vi "RefMem PtByPt RT Driver VI (Async).vi"(6 "Device Clock":string, 9 "Device Inputs FIFO":refnum<k33>, 10 "Device Outputs FIFO":refnum<k33>, 11 "Device Reference":T1 format="%.0x") -> ()   [LabVIEW 2010, in "RefMem PtByPt Custom Device.lvlib"]
uses:
  RefMem PtByPt Custom Device.lvlib
  <vilib>/NI Veristand/Custom Device API/Custom Device Item Ref.ctl
  <vilib>/NI Veristand/Custom Device API/Custom Device Channel Type.ctl
  Controls/Data Channel Type.ctl
  <vilib>/Platform/TimedLoop/XDataNode/XDataNode.xnode
  <vilib>/Platform/TimedLoop/XDataNode/timing_clust.ctl
  <vilib>/Platform/TimedLoop/XDataNode/nitl_modes.ctl
  <vilib>/Platform/TimedLoop/XDataNode/wakeup.ctl
  Controls/Global.vi
  <vilib>/NI Veristand/Custom Device API/Get Item Property (I32).vi
  <vilib>/NI Veristand/Custom Device API/Get Item Property (String).vi
  <vilib>/NI Veristand/Custom Device Tools/Custom Device Utility Library/NI VeriStand - Search for All Items by Property.vi
  <vilib>/NI Veristand/Custom Device API/Get Item Property (U32).vi
  <vilib>/NI Veristand/Custom Device Tools/Custom Device Utility Library/NI VeriStand - Search for Item by Name.vi
  <vilib>/Platform/TimedLoop/XDataNode/XDNodeRunTimeDep.lvlib
  <vilib>/NI Veristand/Custom Device API/Custom Device API.lvlib
  <vilib>/NI Veristand/Custom Device Tools/Custom Device Utility Library/Custom Device Utility Library.lvlib
panel:
  in  "Status Notifier":refnum<notifier>
  # "Custom Device Template\nv1.0"
  # "Use this template as a starting point for creating a custom device code module. The input controls shown here are specially named controls that the system will use to provide the device loop with data. The controls are not required for the device loop to run. For instance, if the device doesn't produce any output data, then you don't need the Device Outputs FIFO control. If you do use these controls, however, they need to have these exact names to be functional."
  # "The optional status notifier element is used to notify the RT engine of the last state of the custom device, and to indicate the device has completed execution. If this control is not used, a default No Error value is returned to the system when the device finishes execution.\n\nNote: This error state is not checked until the system shuts down. Use an output status channel to send more immediate status values to the system."
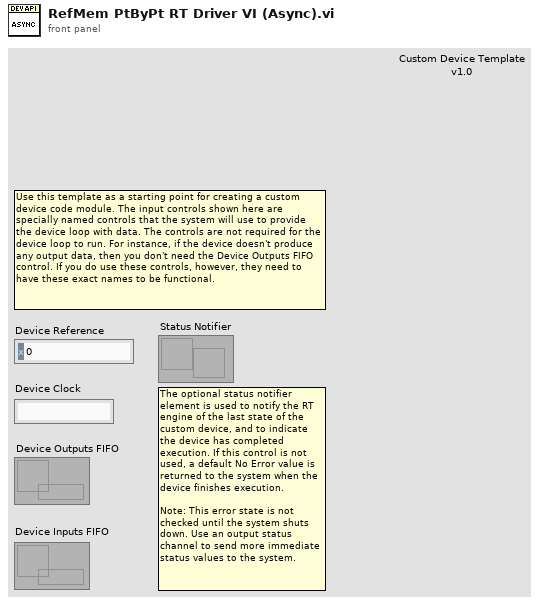
[diagram p1: front panel]
types:
  T1 = typedef "Custom Device API.lvlib/Custom Device Item Ref.ctl" = u64
  T2 = typedef "RefMem PtByPt Custom Device.lvlib/Data Channel Type.ctl" = enum16{"Read", "Write"}
  T3 = typedef "Custom Device API.lvlib/Custom Device Channel Type.ctl" = enum16{"Input", "Output"}
  T4 = typedef "Custom Device API.lvlib/Custom Device Timed Loop Priority.ctl" = enum32{"Low", "Medium", "High"}
  T5 = typedef "XDNodeRunTimeDep.lvlib/timing_clust.ctl" = cluster{"Expected End [f-1]":u64, "Actual End [f-1]":u64, "Finished Late? [f-1]":bool, "Expected End [i-1]":u64, "Actual End [i-1]":u64, "Finished Late? [i-1]":bool, "Expected Start [i]":u64, "Actual Start [i]":u64, "Expected Start [f]":u64, "Actual Start [f]":u64, "Source Name":string, "Structure Name":string, "Period":i64, "Deadline":i64, "Offset":i64, "Start":i64, "Priority":i32, "Timeout":i32, "Mode":T6, "Wakeup Reason":T7, "Error":errorcluster, "Source Type":string, "Secondary Source Type":string, "Global End Time":u64, "Global Start Time":u64, "Frame Duration":u64, "Iteration Duration":u64, "Assigned CPU":i32, "I/O Scan Engine Mode":u32}
  T6 = typedef "XDNodeRunTimeDep.lvlib/nitl_modes.ctl" = enum32{"No Change", "Process missed periods, maintain original phase", "Discard missed periods, maintain original phase", "Process missed periods, ignore original phase", "Discard missed periods, ignore original phase"}
  T7 = typedef "XDNodeRunTimeDep.lvlib/wakeup.ctl" = enum32{"Normal", "Aborted", "Asynchronous wakeup", "Timing source error", "Timed loop error", "Timeout"}
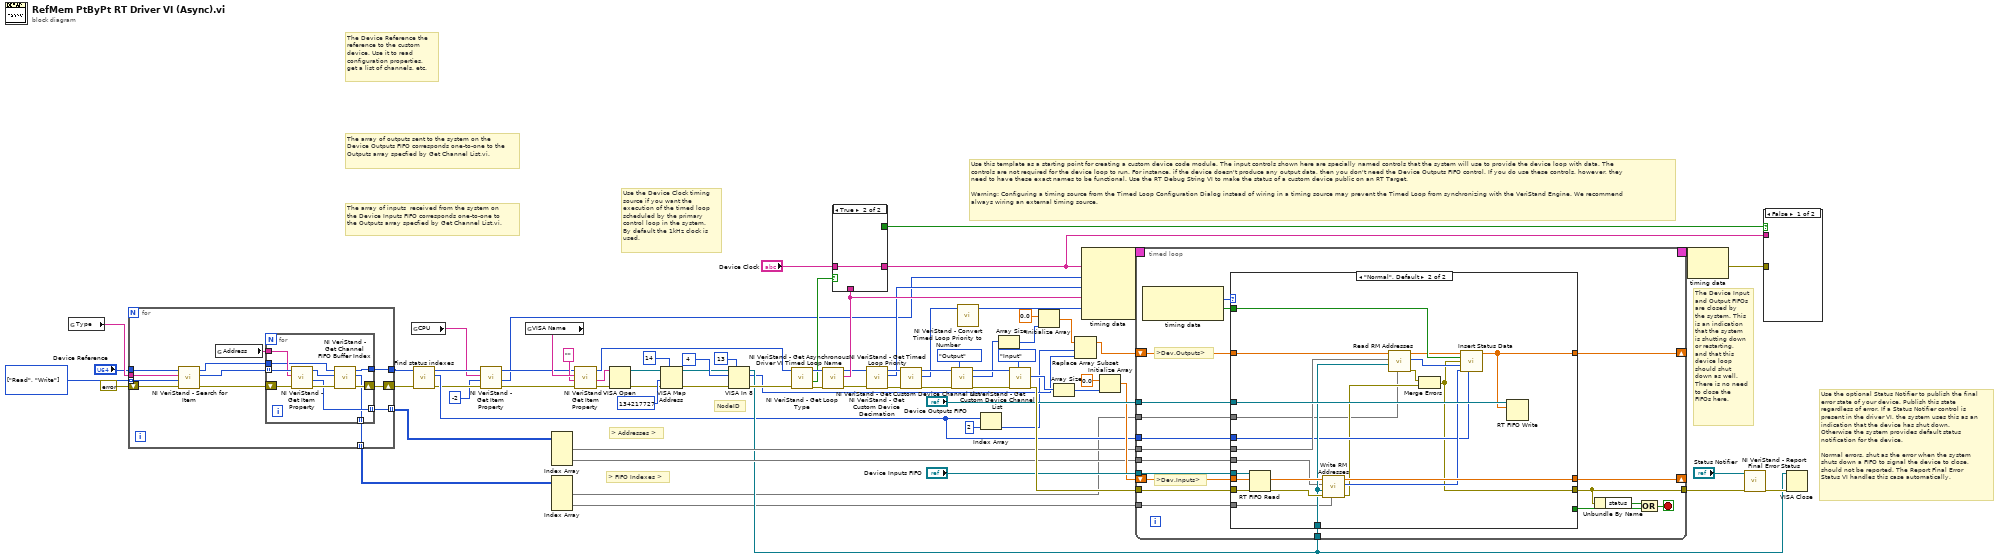
[diagram p0: block diagram]
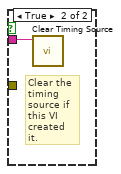
[diagram p2: hidden frame]
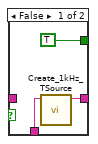
[diagram p3: hidden frame]
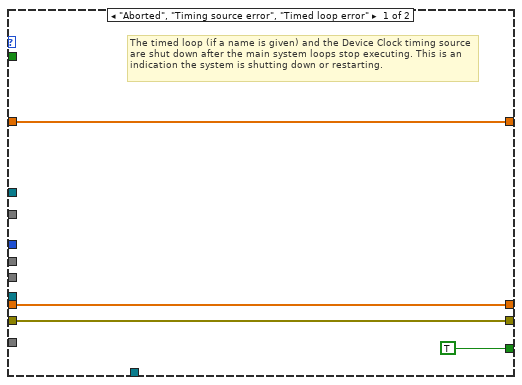
[diagram p4: hidden frame]
diagram:
  w31 = T2[] [enum."Read", enum."Write"] items=["Read", "Write"]
  # "> FIFO Indexes >"
  # "> Addresses >"
  # "NodeID"
  # "The array of inputs  received from the system on the Device Inputs FIFO corresponds one-to-one to the Outputs array specfied by Get Channel List.vi."
  # "Use the optional Status Notifier to publish the final error state of your device. Publish this state regardless of error. If a Status Notifier control is present in the driver VI, the system uses this as an indication that the device has shut down. Otherwise the system provides default status notification for the device.\n\nNormal errors, shut as the error when the system shuts down a FIFO to signal the device to close, should not be reported. The Report Final Error Status VI handles this case automatically."
  # "The Device Input and Output FIFOs are closed by the system. This is an indication that the system is shutting down or restarting, and that this device loop should shut down as well. There is no need to close the FIFOs here."
  # "The array of outputs sent to the system on the Device Outputs FIFO corresponds one-to-one to the Outputs array specfied by Get Channel List.vi."
  # "The Device Reference the reference to the custom device. Use it to read configuration properties, get a list of channels, etc."
  # "Use the Device Clock timing source if you want the execution of the timed loop scheduled by the primary control loop in the system. \nBy default the 1kHz clock is used."
  # "Use this template as a starting point for creating a custom device code module. The input controls shown here are specially named controls that the system will use to provide the device loop with data. The controls are not required for the device loop to run. For instance, if the device doesn't produce any output data, then you don't need the Device Outputs FIFO control. If you do use these controls, however, they need to have these exact names to be functional. Use the RT Debug String VI to make the status of a custom device public on an RT Target.\n\nWarning: Configuring a timing source from the Timed Loop Configuration Dialog instead of wiring in a timing source may prevent the Timed Loop from synchronizing with the VeriStand Engine. We recommend always wiring an external timing source."
  n1 = global read "Global.vi" "Type"() -> (w33:string)
  n2 = for {
    tunnel: w33 -> [w88]
    tunnel: "Device Reference" -> [w87]
    tunnel: w31 -> [w86] mode=indexing
    shift-right: [w81] -> w15
    shift-left: errorcluster {"status"=FALSE, "code"=0, "source"=""} ("error in (no error)") -> [w85]
    tunnel: [w80] -> w29 mode=indexing
    tunnel: [w78] -> w16
    tunnel: [w77] -> w10 mode=indexing
    n3 = call-poly <vilib>:"NI VeriStand - Search for Item.vi"("error in"=w85, "Property Value"=w86, "Property Name"=w88, "Section Ref in"=w87) -> ("error out"=w84:errorcluster, "Item Refs"=w83:T1[], "Section Ref out"=w79:T1)  [unwired: 4 in, 1 out]
    n4 = global read "Global.vi" "Address"() -> (w82:string)
    n5 = for {
      tunnel: w83 -> [w97] mode=indexing
      tunnel: w82 -> [w96]
      shift-right: [w91] -> w81
      shift-left: w84 -> [w98]
      tunnel: [w90] -> w80 mode=indexing
      tunnel: w79 -> [w93]
      tunnel: [w92] -> w78
      tunnel: [w89] -> w77 mode=indexing
      n6 = call-poly <vilib>:"NI VeriStand - Get Item Property.vi"("error in (no error)"=w98, "Property Name"=w96, "Item Ref in"=w97) -> ("error out"=w95:errorcluster, "Value"=w90:u32, "Item Ref out"=w94:T1)  [unwired: 5 in, 1 out]
      n7 = call <vilib>:"NI VeriStand - Get Channel FIFO Buffer Index.vi"("error in"=w95, "Channel Ref"=w94, "Device Ref in"=w93) -> ("error out"=w91:errorcluster, "Channel FIFO Buffer Index"=w89:i32, "Device Ref out"=w92:T1)  [unwired: 4 in, 2 out]
    }
  }
  n8 = global read "Global.vi" "CPU"() -> (w5:string)
  n9 = call "Find status indexes.vi"("error in (no error)"=w15, "Custom Device ref"=w16) -> ("error out"=w6:errorcluster, "Indexes"=w11:i32[], "Custom Device ref"=w7:T1)  [unwired: 7 in]
  n10 = call-poly <vilib>:"NI VeriStand - Get Item Property.vi"("error in (no error)"=w6, "Default Value"=-2 ("Automatic Processor"), "Property Name"=w5, "Item Ref in"=w7) -> ("error out"=w3:errorcluster, "Value"=w1:i32, "Item Ref out"=w2:T1)  [unwired: 4 in, 1 out]
  n11 = global read "Global.vi" "VISA Name"() -> (w43:string)
  n12 = Index Array(array=w29) -> (element #1=w28:u32[], element #2=w27:u32[])  [unwired: 4 in]
  n13 = Index Array(array=w10) -> (element #1=w8:i32[], element #2=w9:i32[])  [unwired: 4 in]
  n14 = call-poly <vilib>:"NI VeriStand - Get Item Property.vi"("error in (no error)"=w3, "Default Value"="", "Property Name"=w43, "Item Ref in"=w2) -> ("error out"=w38:errorcluster, "Value"=w37:string, "Item Ref out"=w35:T1)  [unwired: 4 in, 1 out]
  n15 = VISA Open(error in (no error)=w38, VISA resource name=w37) -> (VISA resource name=w36:refnum<visa-resource-name>, error out=w39:errorcluster)  [unwired: 3 out]
  n16 = VISA Map Address(7:u16 14 ("BAR3"), 8:w39, 9:u32 134217727 ("map size (0)"), 11:w36) -> (0:w24:errorcluster, 3:w23:refnum<visa-resource-name>)  [unwired: 2 in]
  n17 = VISA In 8(7:u16 13 ("BAR2"), 8:w24, 10:u32 4 ("Node ID Register"), 11:w23) -> (0:w22:errorcluster, 2:w18:u8, 3:w21:refnum<visa-resource-name>)
  n18 = call <vilib>:"NI VeriStand - Get Loop Type.vi"("error in (no error)"=w22, "Device Ref in"=w35) -> ("error out"=w58:errorcluster, "Use Device Clock"=w56:bool, "Device Ref out"=w57:T1)  [unwired: 7 out]
  n19 = call <vilib>:"NI VeriStand - Get Asynchronous Driver VI Timed Loop Name.vi"("error in (no error)"=w58, "Device Ref in"=w57) -> ("error out"=w48:errorcluster, "Device Timed Loop Name"=w49:string, "Device Ref out"=w47:T1)  [unwired: 7 out]
  n20 = case shown="True" w56 {
    tunnel: "Device Clock" -> [_ w102]
    tunnel: [w101 w102] -> w50
    tunnel: [TRUE _] -> w51
    tunnel: w49 -> [w99 _]
    frame False {
      n21 = call <vilib>:"Create_1kHz_TSource.vi"("name (in)"=w99) -> ("name (out)"=w101:string)  [unwired: 1 in, 9 out]
    }
    frame True {
    }
  }
  n22 = call <vilib>:"NI VeriStand - Get Custom Device Decimation.vi"("error in (no error)"=w48, "Device Ref in"=w47) -> ("error out"=w45:errorcluster, "Decimation"=w44:i32, "Device Ref out"=w46:T1)  [unwired: 7 in]
  n23 = call <vilib>:"NI VeriStand - Get Timed Loop Priority.vi"("error in (no error)"=w45, "Device Ref in"=w46) -> ("error out"=w63:errorcluster, "Priority"=w61:T4, "Device Ref out"=w64:T1)  [unwired: 7 out]
  n24 = call <vilib>:"NI VeriStand - Get Custom Device Channel List.vi"("Channel Type"=Custom_Device_Channel_Type."Output", "error in (no error)"=w63, "Device Ref in"=w64) -> ("error out"=w66:errorcluster, "Specified Channel Ref List"=w12:T1[], "Device Ref out"=w67:T1)  [unwired: 6 out]
  n25 = call <vilib>:"NI VeriStand - Convert Timed Loop Priority to Number.vi"("Priority"=w61) -> ("Numeric Priority"=w60:i32)  [unwired: 10 out]
  n26 = Index Array(array=w11, index=2) -> (element=w13:i32)
  n27 = Array Size(array=w12) -> (size(s)=w17:i32)
  n28 = call <vilib>:"NI VeriStand - Get Custom Device Channel List.vi"("Channel Type"=Custom_Device_Channel_Type."Input", "error in (no error)"=w66, "Device Ref in"=w67) -> ("error out"=w76:errorcluster, "Specified Channel Ref List"=w62:T1[])  [unwired: 7 out]
  n29 = Initialize Array(0.0 ("element"), w17) -> (w20:dbl[])
  n30 = Array Size(array=w62) -> (size(s)=w59:i32)
  n31 = Replace Array Subset(array=w20, new element=w18, index=w13) -> (w19:dbl[])
  n32 = node-c288(w50, w1, w44, w49, w60) -> (w73:T5)
  n33 = Initialize Array(0.0 ("element"), w59) -> (w69:dbl[])
  n34 = timed-loop {
    timing: w73 -> [_]
    timing-out: [_] -> w72
    shift-right: [w119] -> _
    shift-left: w69 -> [w120]
    shift-right: [w116] -> _
    shift-left: w19 -> [w117]
    tunnel: "Device Outputs FIFO" -> [w115]
    tunnel: "Device Inputs FIFO" -> [w114]
    tunnel: w76 -> [w121]
    tunnel: [w113] -> w53
    tunnel: w21 -> [w108]
    tunnel: w28 -> [w107]
    tunnel: w27 -> [w106]
    tunnel: w11 -> [w105]
    tunnel: w9 -> [w104]
    tunnel: w8 -> [w103]
    stop <- w110 stop-if-true
    # ">Dev.Outputs>"
    # ">Dev.Inputs>"
    n35 = node-c288() -> (w118:T7, w109:bool)  [unwired: 1 out]
    n36 = case shown="\"Normal\", Default" w118 {
      tunnel: w121 -> [w124 w142]
      tunnel: w120 -> [w125 w144]
      tunnel: [w124 w128] -> w113
      tunnel: [w125 w141] -> w119
      tunnel: w117 -> [w123 w145]
      tunnel: [w123 w143] -> w116
      tunnel: w115 -> [_ w147]
      tunnel: w114 -> [_ w146]
      tunnel: [TRUE _] -> w111
      tunnel: w109 -> [_ w137]
      tunnel: w108 -> [_ w136]
      tunnel: w107 -> [_ w133]
      tunnel: w106 -> [_ w132]
      tunnel: w105 -> [_ w131]
      tunnel: w104 -> [_ w127]
      tunnel: w103 -> [_ w126]
      frame "Aborted", "Timing source error", "Timed loop error" {
        # "The timed loop (if a name is given) and the Device Clock timing source are shut down after the main system loops stop executing. This is an indication the system is shutting down or restarting."
      }
      frame "Normal", Default {
        n37 = RT FIFO Read(0:w146, 1:w144, 3:w142) -> (9:w140:dbl[], 11:w139:errorcluster)  [unwired: 4 out]
        n38 = call "Write RM Addresses.vi"("FIFO Idxs"=w127, "error in"=w139, "Session"=w136, "Addresses"=w132, "Values"=w140) -> ("error out"=w129:errorcluster, "Write Duration"=w138:u32, "Values"=w141:dbl[])  [unwired: 4 in]
        n39 = call "Read RM Addresses.vi"("FIFO Idxs"=w126, "Session"=w136, "Addresses"=w133, "Old Values"=w145) -> ("error out"=w130:errorcluster, "Read Duration"=w134:u32, "Updated Values"=w135:dbl[])  [unwired: 5 in]
        n40 = Merge Errors(w130, w129) -> (w128:errorcluster)
        n41 = call "Insert Status Data.vi"("OutputData in"=w135, "Late?"=w137, "error in (no error)"=w128, "Read Duration"=w134, "Write Duration"=w138, "Status Channel Indexes"=w131) -> ("OutputData out"=w143:dbl[])  [unwired: 9 in]
        n42 = RT FIFO Write(0:w147, 1:w143) -> ()  [unwired: 2 in, 5 out]
      }
    }
    n43 = Unbundle By Name(w113) -> ("status"=w112:bool)
    n44 = Compound Arithmetic op=OR(w112, w111) -> (w110:bool)
  }
  n45 = node-c288(w72) -> (w52:errorcluster)
  n46 = call <vilib>:"NI VeriStand - Report Final Error Status.vi"("error in (no error)"=w53, "Status Notifier"="Status Notifier") -> ("error out"=w34:errorcluster)  [unwired: 1 in, 8 out]
  n47 = case shown="False" w51 {
    tunnel: w52 -> [_ _]
    tunnel: w50 -> [_ w152]
    frame False {
    }
    frame True {
      # "Clear the timing source if this VI created it."
      n48 = call <vilib>:"Clear Timing Source.vi"("name"=w152) -> ()  [unwired: 1 in, 10 out]
    }
  }
  n49 = VISA Close(VISA resource name=w21, error in (no error)=w34) -> ()  [unwired: 1 out]
